vi "MHM Write Register I2C Ex.vi"(6 "pulValid":u32[](array[numeric]), 7 "pulData":u32[](array[numeric]), 8 "error in (no error)":errorcluster, 9 "ulI2CSlaveAdr":u32, 10 "ulArraySize":u32, 11 "ulMHMHandle":u32) -> (0 "error out (no error)":errorcluster, 3 "function return":u32)   [LabVIEW 2017, in "MHM_1SL_interface.lvlib"]
uses:
  MHM_1SL_interface.lvlib
  SSI_Tool/DUT_Interface/lv_interface/lib/MHM_1SL_interface.dll
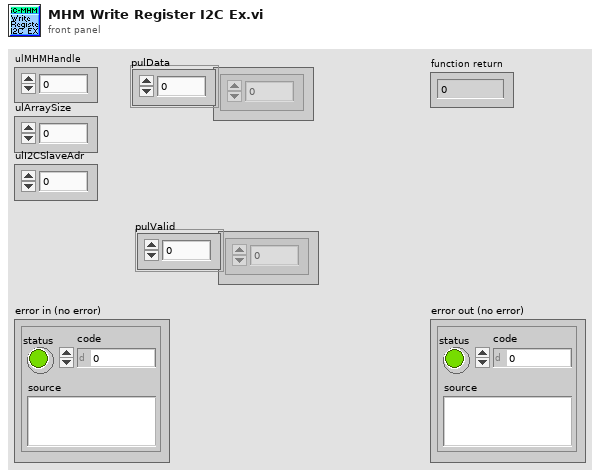
[diagram p1: front panel]
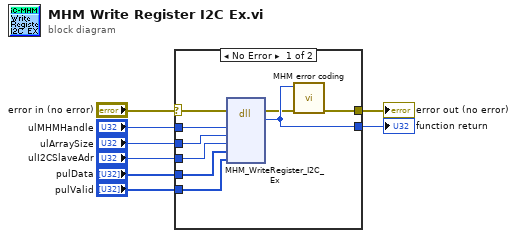
[diagram p0: block diagram]
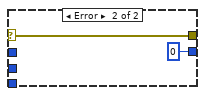
[diagram p2: hidden frame]
diagram:
  n1 = case shown="No Error" "error in (no error)" {
    selector: "error in (no error)" -> [w13 w19]
    tunnel: [w17 u32 0] -> w8
    tunnel: "ulMHMHandle" -> [w16 _]
    tunnel: [w14 w19] -> w6
    tunnel: "ulArraySize" -> [w12 _]
    tunnel: "ulI2CSlaveAdr" -> [w11 _]
    tunnel: "pulData" -> [w10 _]
    tunnel: "pulValid" -> [w9 _]
    frame No Error {
      n2 = dll-call lib="C:/workspace/project/scancon/sw/SSI_Tool/DUT_Interface/lv_interface/lib/MHM_1SL_interface.dll" fn="MHM_WriteRegister_I2C_Ex"(error in=w13, "ulMU150Handle"=w16, "ulArraySize"=w12, "ulI2CSlaveAdr"=w11, "pulData"=w10, "pulValid"=w9) -> (error out=w15:errorcluster, "return type"=w17:u32)  [unwired: 7 in, 1 out]
      n3 = call "MHM error coding.vi"("error in (no error)"=w15, "function return in"=w17) -> ("error out"=w14:errorcluster)  [unwired: 9 in]
    }
    frame Error {
    }
  }
  "function return" <- w8
  "error out (no error)" <- w6
